vi "Write Temperature.vi"(8 "error in (no error)":errorcluster, 10 "Temperature":dbl, 11 "CCDCamera in":refnum<class "CCDCamera.lvclass">) -> (0 "error out":errorcluster, 3 "CCDCamera out":refnum<class "CCDCamera.lvclass">)   [LabVIEW 2018, in "CCDCamera.lvclass"]
doc: "This VI sets the CCD temperature."
uses:
  CCDCamera.lvclass
  CCDCamera.lvclass/CCDCamera.ctl
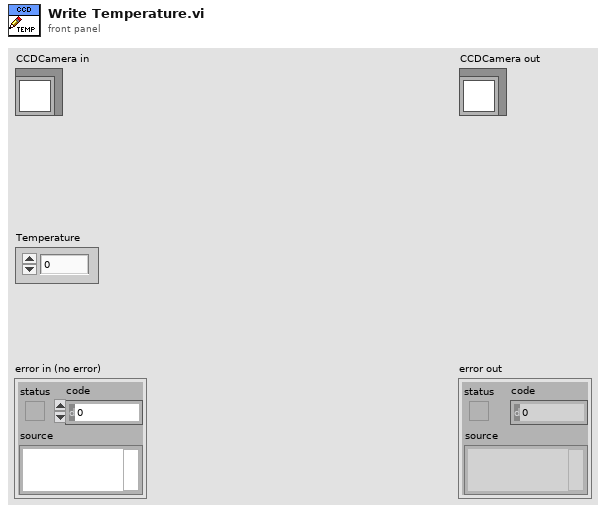
[diagram p1: front panel]
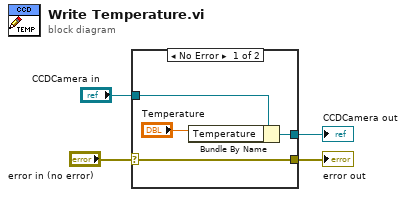
[diagram p0: block diagram]
diagram:
  n1 = case shown="No Error" "error in (no error)" {
    selector: "error in (no error)" -> [w6 w10]
    tunnel: [w6 w10] -> w3
    tunnel: [w7 w9] -> w1
    tunnel: "CCDCamera in" -> [w8 w9]
    frame No Error {
      n2 = Bundle By Name(cluster=w8, "Temperature"="Temperature") -> (w7:refnum<class "CCDCamera.lvclass">)
    }
    frame Error {
    }
  }
  "error out" <- w3
  "CCDCamera out" <- w1
